vi "onStop.vi"(8 "error in (no error)":errorcluster, 11 "SMO":refnum<class "SMO.lvclass">) -> (0 "error out":errorcluster, 3 "SMO out":refnum<class "SMO.lvclass">)   [LabVIEW 2013, in "SMO.lvclass"]
uses:
  SMO.lvclass
  SMO.lvclass/SMO.ctl
  Typedefs/SMO Dependency--Cluster.ctl
  Support/Attribute.Owner/Attribute.Owner.lvclass
panel:
  # "For instructions on how to use the JKI State Machine Objects, examples and video tutorials, visit:\nhttp://jki.net/state-machine-objects/\n\nJKI State Machine Objects™\nhttp://jki.net/state-machine-objects/\nCopyright (C) 2005-2015, JKI <info@jki.net>\nALL RIGHTS RESERVED"
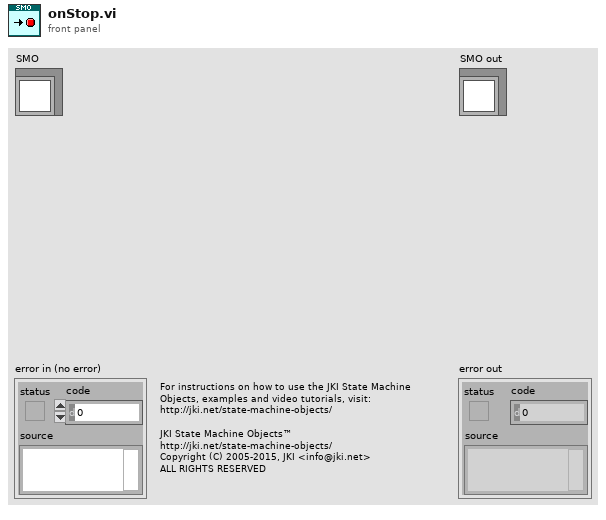
[diagram p1: front panel]
types:
  T1 = typedef "SMO.lvclass/SMO Dependency--Cluster.ctl" = cluster{"Dependency":refnum<class "SMO.lvclass">, "Level":string}
  T2 = typedef "SMO.lvclass/PrivateData--Ref.ctl" = refnum<data-value>
  T3 = typedef "SMO.lvclass/PrivateData--Cluster.ctl" = cluster{"Parent Call":T4, "Registered Processes":T5[], "Sync Notifier":refnum<notifier>, "Process Error Notifier":refnum<notifier>, "Protected Events":T6, "Public Events":T7, "SMO State":T8, "[Dependencies]":T1[], "[Attributes]":refnum<class "Attribute.lvclass">[], "Launcher Close":refnum<notifier>}
  T4 = typedef "SMO.lvclass/Parent Call--Enum.ctl" = enum16{"Allows parent to run", "Does not request parent to run"}
  T5 = typedef "SMO.lvclass/RegisteredProcessData--Cluster.ctl" = cluster{"Name":string, "Static VI Ref":refnum<vi>, "Running":bool, "NotifierRef":u32}
  T6 = typedef "SMO.lvclass/Protected Events.ctl" = cluster{"StopProcesses":refnum<user-event>, "AbortProcesses":refnum<user-event>, "Config Changed":refnum<user-event>}
  T7 = typedef "SMO.lvclass/Public Events.ctl" = cluster{"Error":refnum<user-event>, "State":refnum<user-event>}
  T8 = typedef "SMO.lvclass/SMOState --Enum.ctl" = enum16{"unknown", "Created", "Started", "Stopped"}
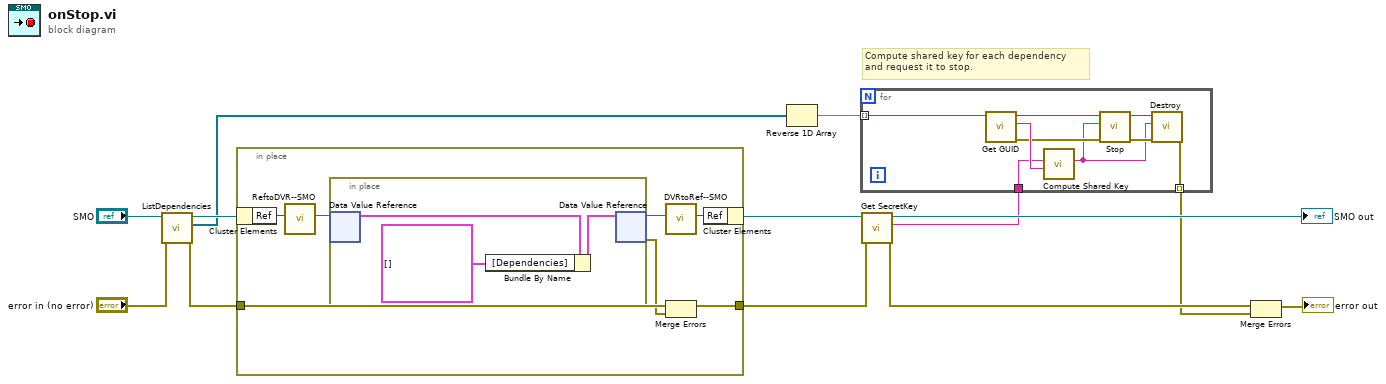
[diagram p0: block diagram]
diagram:
  # "Compute shared key for each dependency\nand request it to stop."
  n1 = call "ListDependencies.vi"("error in (no error)"="error in (no error)", "SMO in"="SMO") -> ("error out"=w2:errorcluster, "[Dependencies]"=w1:refnum<class "SMO.lvclass">[], "SMO out"=w4:refnum<class "SMO.lvclass">)  [unwired: 6 in, 1 out]
  n2 = in-place {
    in-place-border: w2 -> [w16]
    in-place-border: [w14] -> w11
    n3 = in-place-cluster #1(w4) -> ("Ref"=w20:u32)
    n4 = call "ReftoDVR--SMO.vi"("Ref"=w20) -> ("Ref"=w19:T2)  [unwired: 10 in]
    n5 = in-place {
      n6 = in-place-dvr #2(w19) -> (w23:T3)  [unwired: 1 out]
      n7 = Bundle By Name(cluster=w23, "[Dependencies]"=T1[] []) -> (w22:T3)
      n8 = in-place-dvr #2(w22) -> (w18:T2, w15:errorcluster)
    }
    n9 = call "DVRtoRef--SMO.vi"("Ref"=w18) -> ("Ref"=w17:u32)  [unwired: 10 in]
    n10 = Merge Errors(w16, w15) -> (w14:errorcluster)
    n11 = in-place-cluster #1("Ref"=w17) -> (w6:refnum<class "SMO.lvclass">)
  }
  n12 = Reverse 1D Array(array=w1) -> (reversed array=w9:refnum<class "SMO.lvclass">[])
  n13 = call "Get SecretKey.vi"("error in (no error)"=w11, "SMO"=w6) -> ("error out"=w12:errorcluster, "SecretKey"=w10:string, "SMO out"=→"SMO out":refnum<class "SMO.lvclass">)  [unwired: 7 in]
  n14 = for {
    tunnel: w9 -> [w24] mode=indexing
    tunnel: w10 -> [w30]
    tunnel: [w25] -> w8 mode=indexing
    n15 = call "Get GUID.vi"("SMO"=w24) -> ("error out"=w29:errorcluster, "GUID"=w31:string, "SMO out"=w32:refnum<class "SMO.lvclass">)  [unwired: 8 in]
    n16 = call "Compute Shared Key.vi"("GUID"=w31, "SecretKey"=w30) -> ("Shared Key"=w26:string)  [unwired: 9 in]
    n17 = call "Stop.vi"("error in (no error)"=w29, "Shared Key"=w26, "SMO"=w32) -> ("error out"=w27:errorcluster, "SMO out"=w28:refnum<class "SMO.lvclass">)  [unwired: 7 in]
    n18 = call "Destroy.vi"("error in (no error)"=w27, "Shared Key"=w26, "SMO"=w28) -> ("error out"=w25:errorcluster)  [unwired: 8 in]
  }
  n19 = Merge Errors(w12, w8) -> (→"error out":errorcluster)
